vi "Temp Report.vi"   [LabVIEW 2020]
uses:
  Report.lvlib
  Test Setting.ctl
  REP Configuration.ctl
types:
  T1 = typedef "Report.lvlib/REP Configuration.ctl" = cluster{"Test Setting":T2, "Measurements":string[][], "LOG REF":refnum<vi>, "GAGES Configuration":cluster{"Type":string, "LOT":string, "WO":string, "Over Coat":string, "STC":string, "Description":string, "Foil":string, "GL":string, "GW":string, "Resistance":dbl}, "Report Template":path, "Save Report path":path, "Data File Path":path, "Popup Dialog":bool}
  T2 = typedef "Report.lvlib/Test Setting.ctl" = cluster{"Test_Num":i32, "Test_ID":i32, "Proc_ID":i32, "Max Force":dbl, "User":string, "SN":string, "Date":string}
  T3 = typedef "Report.lvlib/REP Configuration.ctl" = cluster{"Test Setting":T2, "Measurements":string[][], "LOG REF":refnum<vi>, "Report Template":path, "Save Report path":path, "Data File Path":path, "Popup Dialog":bool}
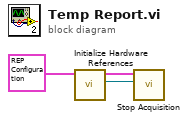
[diagram p0: block diagram]
diagram:
  n1 = call "Initialize Hardware References.vi"("Hardware Resources in"=T1 {"Test Setting"={"Test_Num"=0, "Test_ID"=0, "Proc_ID"=0, "Max Force"=0.0, "User"="", "SN"="", "Date"=""}, "Measurements"=[[""]], "LOG REF"=refnum, "GAGES Configuration"={"Type"="", "LOT"="", "WO"="", "Over Coat"="", "STC"="", "Description"="", "Foil"="", "GL"="", "GW"="", "Resistance"=0.0}, "Report Template"=path "D:/Dropbox/Work/Vishay/FTS/SW Code/Report template.xltm", "Save Report path"=path "D:/Dropbox/Work/Vishay/FTS/SW Code/Excel report", "Data File Path"=path "", "Popup Dialog"=TRUE}) -> ("report out"=w2:refnum<class "NI_report.lvclass">, "Hardware Resources out"=w3:T3)  [unwired: 8 in, 1 out]
  n2 = call "Stop Acquisition.vi"("report in"=w2, "Hardware Resources in"=w3) -> ()  [unwired: 9 in, 1 out]
